vi "factorial.vi"() -> ()   [LabVIEW 2019]
panel:
  out "factorial":i32
  in  "Number":i32
  # "Factorial of Number"
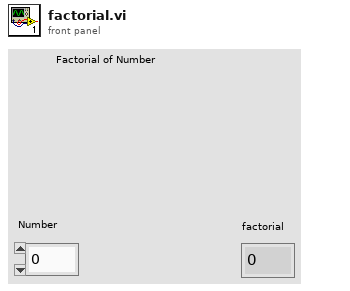
[diagram p1: front panel]
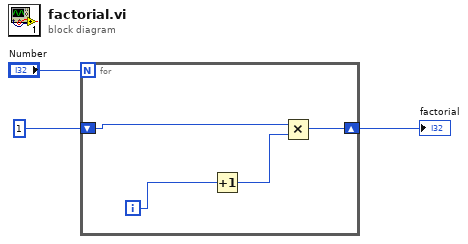
[diagram p0: block diagram]
diagram:
  n1 = for {
    N: "Number" -> [_]
    shift-right: [w4] -> w1
    shift-left: 1 -> [w7]
    i -> [w6]
    n2 = Increment(x=w6) -> (x+1=w5:i32)
    n3 = Multiply(x=w7, y=w5) -> (x*y=w4:i32)
  }
  "factorial" <- w1
